vi "main.vi"() -> ()   [LabVIEW 2024]
uses:
  StateVariable.ctl
panel:
  out "Waveform Chart":T1(graph)
  out "State name":string
  in  "Stop":bool
  # "Template : LabVIEW  State Machine Basic"
  # "LINE: THAITECHZONE"
  # "Signal Acquired"
  # "State"
  # "NATTAPHOL JASUNGNUEN"
  # "LINE : @thaitechzone"
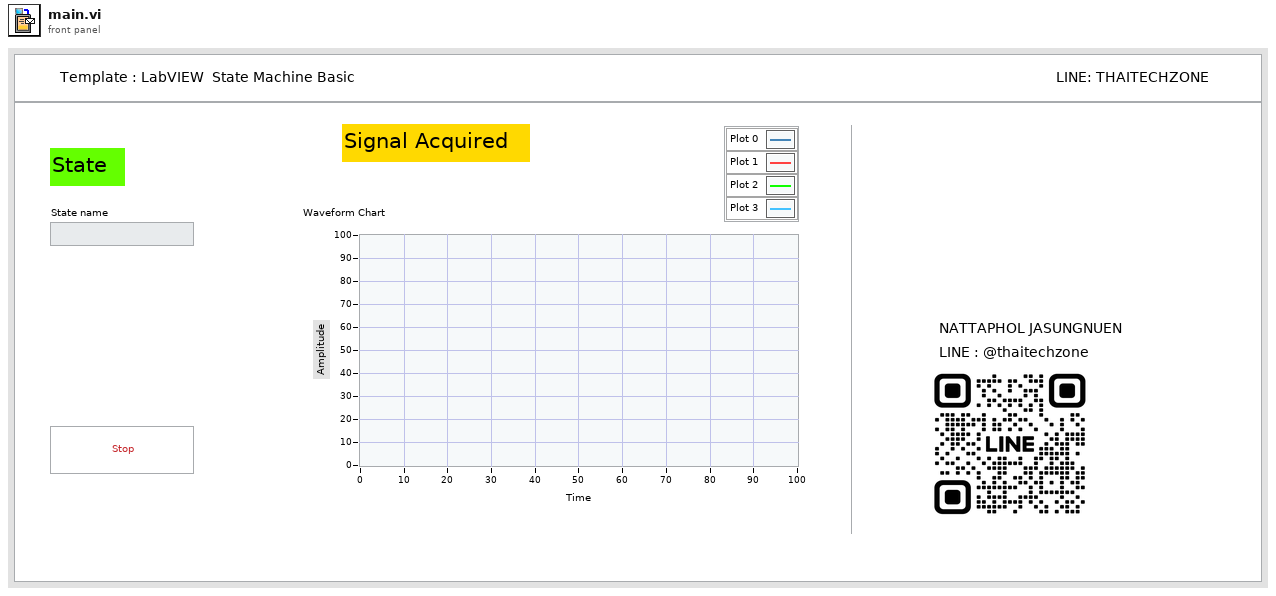
[diagram p1: front panel]
types:
  T1 = cluster{"Array Out[0]":u64, "Array Out[1]":u64, "Array Out[2]":u64, "Array Out[3]":u64, "Array Out[4]":u64, "Array Out[5]":u64, "Array Out[6]":u64, "Array Out[7]":u64, "Array Out[8]":u64}
  T2 = typedef "StateVariable.ctl" = enum16{"Initialization", "Acquired Data", "Processing", "Logging", "Update  Display Data"}
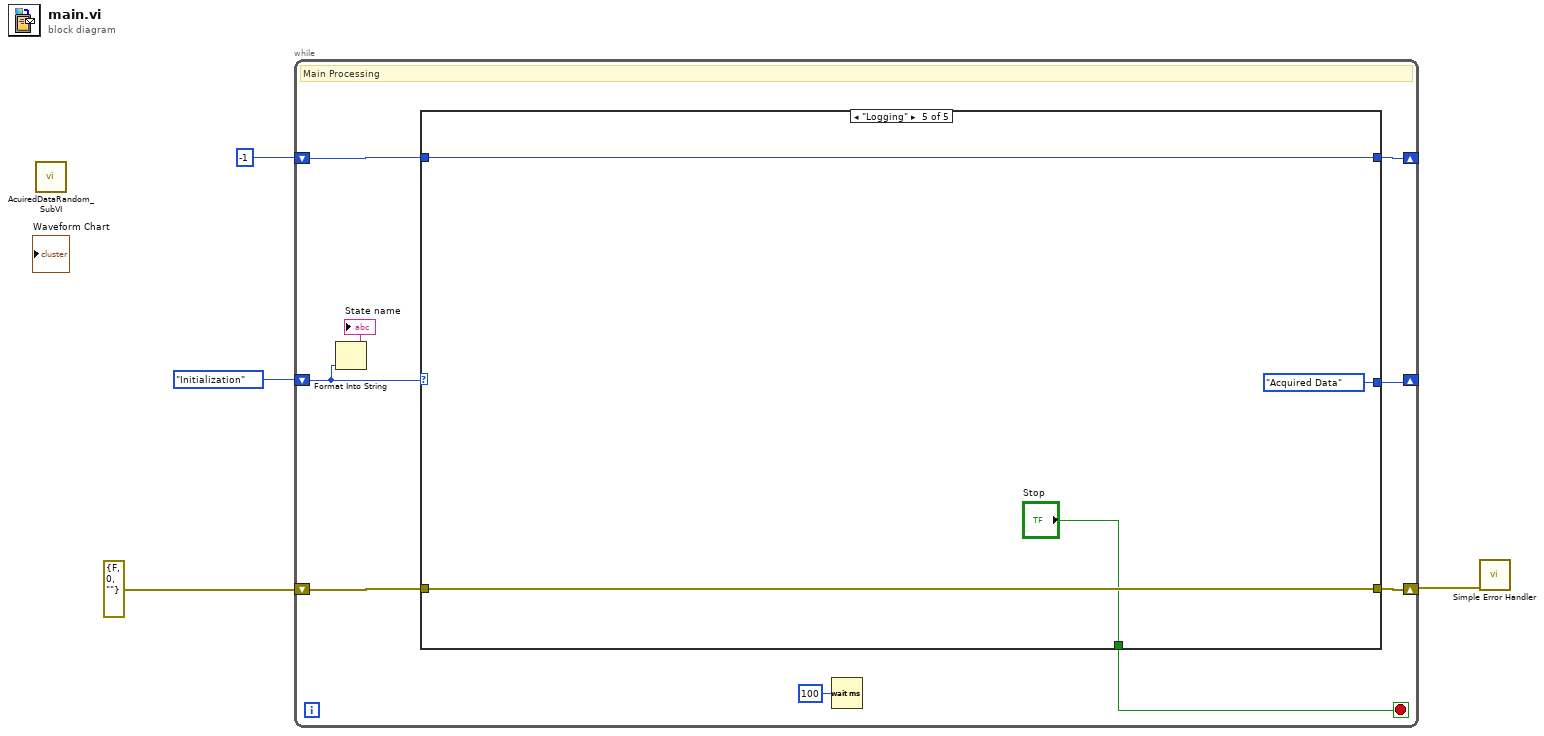
[diagram p0: block diagram]
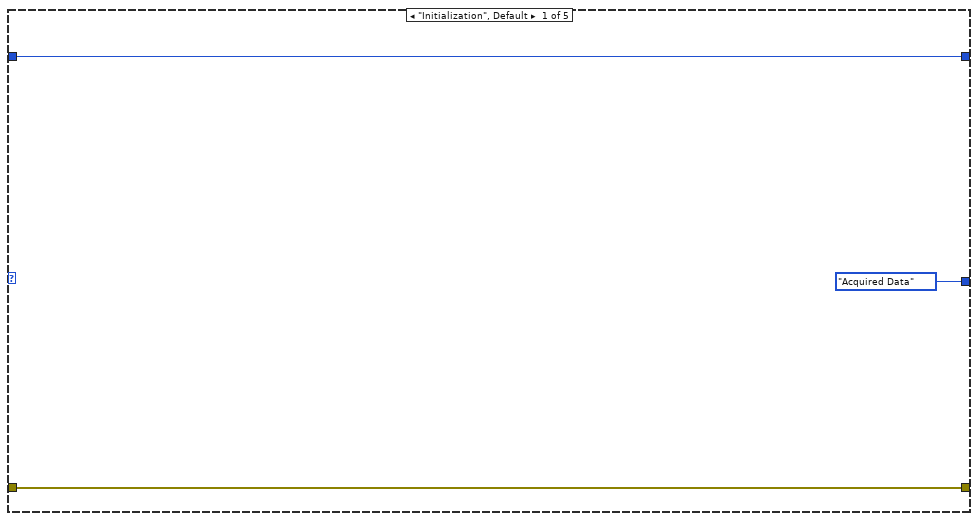
[diagram p2: hidden frame]
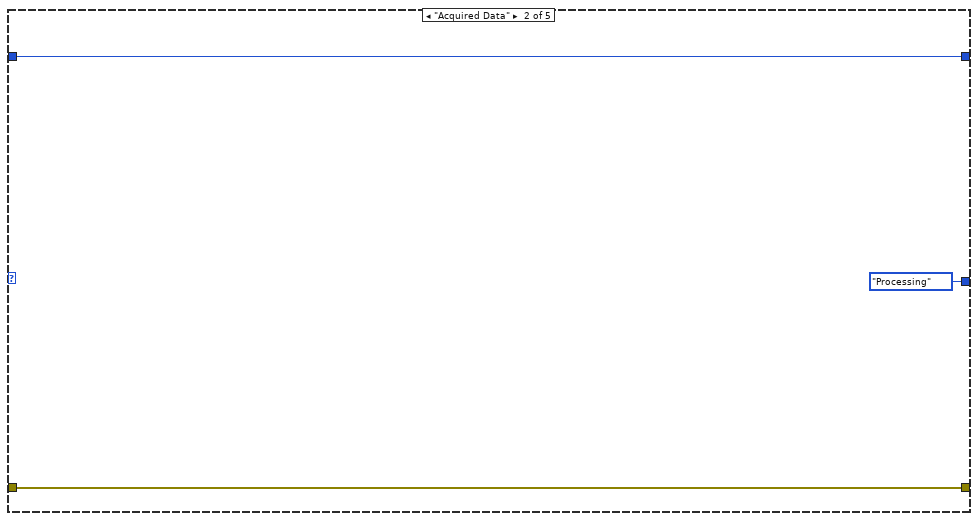
[diagram p3: hidden frame]
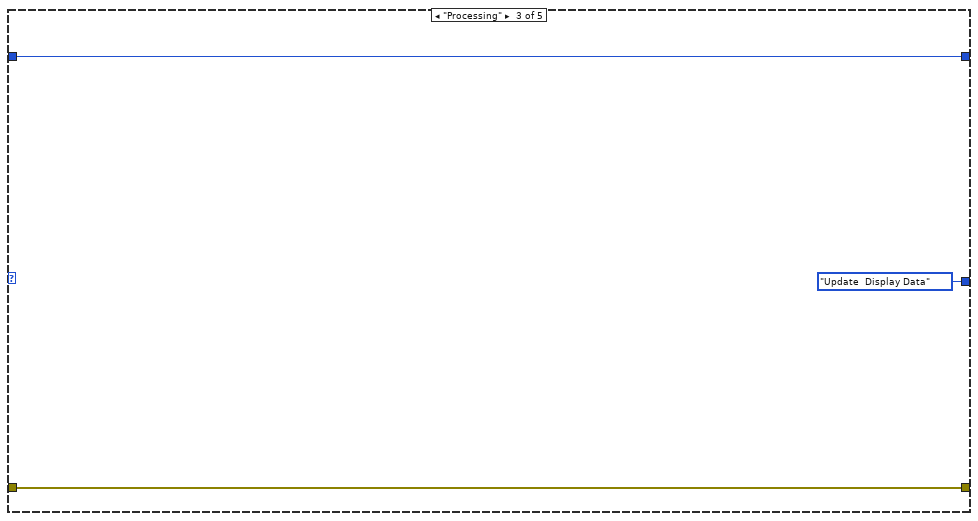
[diagram p4: hidden frame]
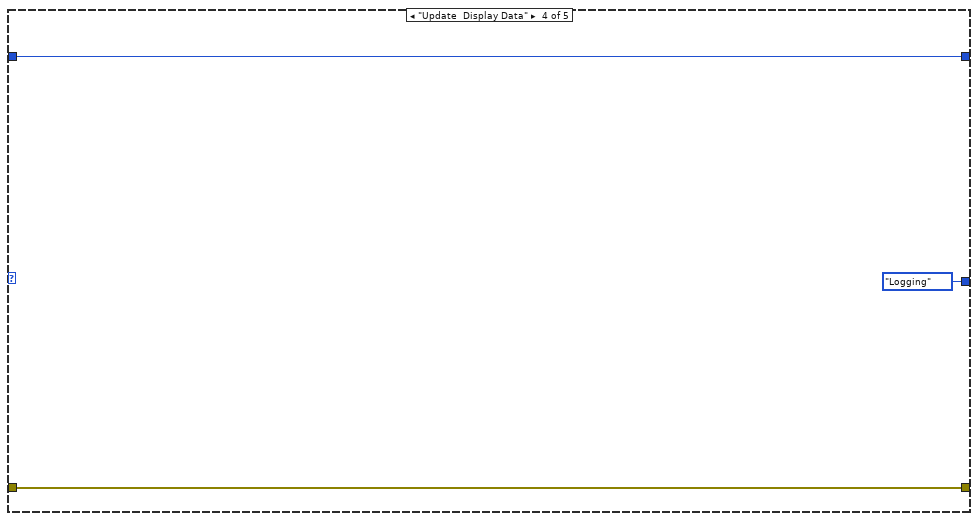
[diagram p5: hidden frame]
diagram:
  n1 = call "AcuiredDataRandom_SubVI.vi"() -> ()  [unwired: 11 in, 1 out]
  n2 = while {
    shift-right: [w7] -> _
    shift-left: StateVariable."Initialization" ("Enum") -> [w6]
    shift-right: [w10] -> _
    shift-left: -1 -> [w11]
    shift-right: [w8] -> w3
    shift-left: errorcluster {"status"=FALSE, "code"=0, "source"=""} ("error constant") -> [w9]
    stop <- w5 stop-if-true
    # "Main Processing"
    n3 = Format Into String(w6) -> (resulting string=→"State name":string)  [unwired: 3 in, 1 out]
    n4 = case shown="\"Logging\"" w6 {
      tunnel: w11 -> [w16 w19 w22 w25 w29]
      tunnel: [w16 w19 w22 w25 w29] -> w10
      tunnel: w9 -> [w15 w18 w21 w24 w28]
      tunnel: [w15 w18 w21 w24 w28] -> w8
      tunnel: [StateVariable."Acquired Data" ("Enum") StateVariable."Processing" ("Enum") StateVariable."Update  Display Data" ("Enum") StateVariable."Logging" ("Enum") StateVariable."Acquired Data" ("Enum")] -> w7
      tunnel: [_ _ _ _ "Stop"] -> w5
      frame "Initialization", Default {
      }
      frame "Acquired Data" {
      }
      frame "Processing" {
      }
      frame "Update  Display Data" {
      }
      frame "Logging" {
      }
    }
    n5 = Wait (ms)(milliseconds to wait=u32 100) -> ()  [unwired: 1 out]
  }
  n6 = call <vilib>:"Simple Error Handler.vi"("error in (no error)"=w3) -> ()  [unwired: 4 in, 5 out]
